vi "Sequence Init.vi"(8 "error in (no error)":errorcluster, 11 "MSX-E3711 in":refnum<class "MSX-E3711.lvclass">) -> (0 "error out":errorcluster, 3 "MSX-E3711 out":refnum<class "MSX-E3711.lvclass">)   [LabVIEW 2014, in "MSX-E3711.lvlib" / "MSX-E3711.lvclass"]
uses:
  MSX-E3711.lvclass
  DriverMasterSync/build/DriverMasterSync.lvlibp/Modules/HAL/DriverMasterSync/DriverMasterSyncClass/DriverMasterSync.lvclass
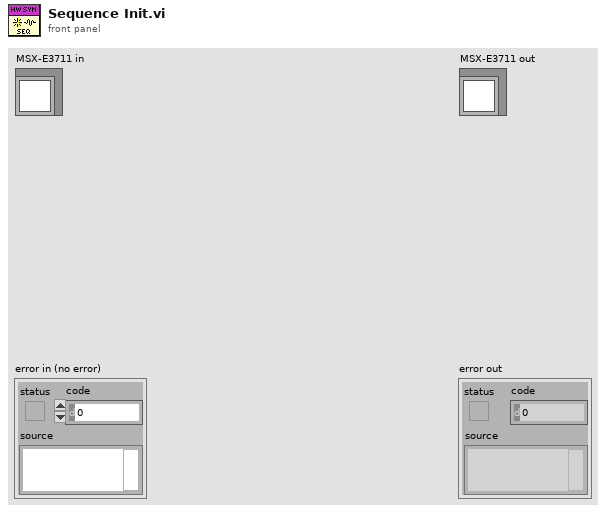
[diagram p1: front panel]
types:
  T1 = typedef "DriverMasterSync.lvlibp/HAL Config Data.ctl" = cluster{"HWSync Index":u32, "Driver Name":string, "Channel Mask":u64}
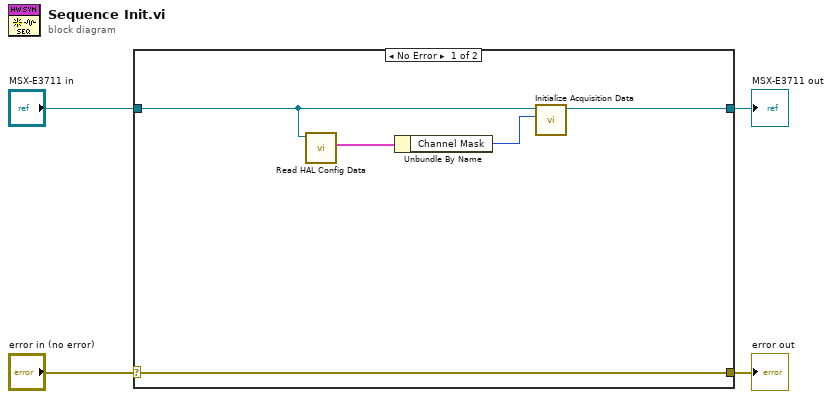
[diagram p0: block diagram]
diagram:
  n1 = case shown="No Error" "error in (no error)" {
    selector: "error in (no error)" -> [w5 w11]
    tunnel: [w5 w11] -> w3
    tunnel: [w7 w10] -> w1
    tunnel: "MSX-E3711 in" -> [w6 w10]
    frame No Error {
      n2 = call "Read HAL Config Data.vi"("DriverMasterSync in"=w6) -> ("HAL Config Data"=w9:T1)  [unwired: 8 in, 2 out]
      n3 = Unbundle By Name(w9) -> ("Channel Mask"=w8:u64)
      n4 = call "Initialize Acquisition Data.vi"("Channel Mask"=w8, "DriverMasterSync in"=w6) -> ("DriverMasterSync out"=w7:refnum<class "MSX-E3711.lvclass">)  [unwired: 8 in, 1 out]
    }
    frame Error {
    }
  }
  "error out" <- w3
  "MSX-E3711 out" <- w1
